vi "Delete Item from LVClass.vi"(7 "Item Type":string="VI", 8 "error in (no error)":errorcluster, 10 "Item name":string, 11 "LVClassLibrary in":refnum<vi>) -> (0 "error out":errorcluster, 2 "Deleted ?":bool, 3 "LVClassLibrary out":refnum<vi>)   [LabVIEW 2019, in "gRPC Template Creation Utility.lvlib"]
uses:
  gRPC Template Creation Utility.lvlib
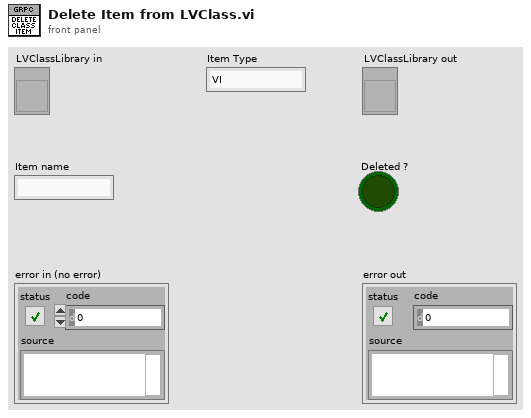
[diagram p1: front panel]
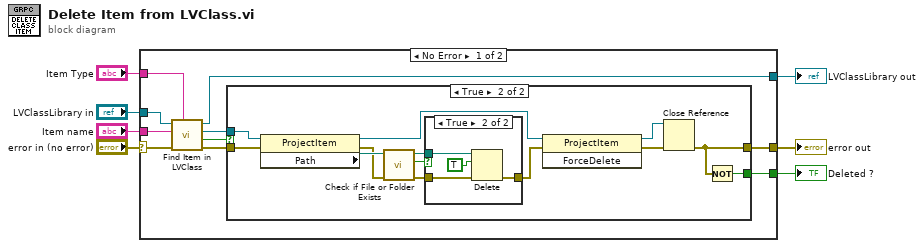
[diagram p0: block diagram]
diagram:
  n1 = case shown="No Error" "error in (no error)" {
    selector: "error in (no error)" -> [w10 w38]
    tunnel: [w17 w37] -> w7
    tunnel: "Item name" -> [w16 _]
    tunnel: "LVClassLibrary in" -> [w15 w37]
    tunnel: "Item Type" -> [w14 _]
    tunnel: [w9 w38] -> w2
    tunnel: [w8 _] -> w1
    frame No Error {
      n2 = call "Find Item in LVClass.vi"("Item Type"=w14, "error in (no error)"=w10, "Item Name"=w16, "Class Item in"=w15) -> ("error out"=w11:errorcluster, "Found?"=w13:bool, "Project Item (Class Item)"=w12:refnum<vi>, "Class Item out"=w17:refnum<vi>)  [unwired: 4 in]
      n3 = case shown="True" w13 {
        tunnel: w12 -> [_ w31]
        tunnel: w11 -> [w18 w27]
        tunnel: [w18 w19] -> w9
        tunnel: [_ w30] -> w8
        frame False {
        }
        frame True {
          n4 = property class="ProjectItem"(reference=w31, error in=w27) -> (reference out=w28:refnum<vi>, error out=w25:errorcluster, "Path"=w26:path)
          n5 = call <vilib>:"Check if File or Folder Exists.vi"("error in (no error)"=w25, "path"=w26) -> ("error out"=w23:errorcluster, "file or folder exists?"=w29:bool, "dup path"=w24:path)  [unwired: 7 in]
          n6 = case shown="True" w29 {
            tunnel: w24 -> [_ w36]
            tunnel: w23 -> [w32 w35]
            tunnel: [w32 w34] -> w22
            frame False {
            }
            frame True {
              n7 = Delete(path (use dialog)=w36, entire hierarchy (F)=TRUE, error in=w35) -> (error out=w34:errorcluster)  [unwired: 2 in, 2 out]
            }
          }
          n8 = invoke class="ProjectItem" method="ForceDelete"(reference=w28, error in=w22) -> (reference out=w20:refnum<vi>, error out=w21:errorcluster)  [unwired: 1 in, 1 out]
          n9 = Close Reference(reference=w20, error in (no error)=w21) -> (error out=w19:errorcluster)
          n10 = Not(x=w19) -> (.not. x?=w30:bool)
        }
      }
    }
    frame Error {
    }
  }
  "LVClassLibrary out" <- w7
  "error out" <- w2
  "Deleted ?" <- w1
